vi "stage_move_absolute.vi"(7 "Stage Name":string, 8 "error in (no error)":errorcluster, 9 "wait_for_done":bool, 10 "Position":dbl, 11 "newport_xps in":refnum<class "newport_xps.lvclass">) -> (0 "error out":errorcluster, 3 "newport_xps out":refnum<class "newport_xps.lvclass">)   [LabVIEW 2015, in "newport_xps.lvclass"]
uses:
  newport_xps.lvclass
  newport_xps.lvclass/newport_xps.ctl
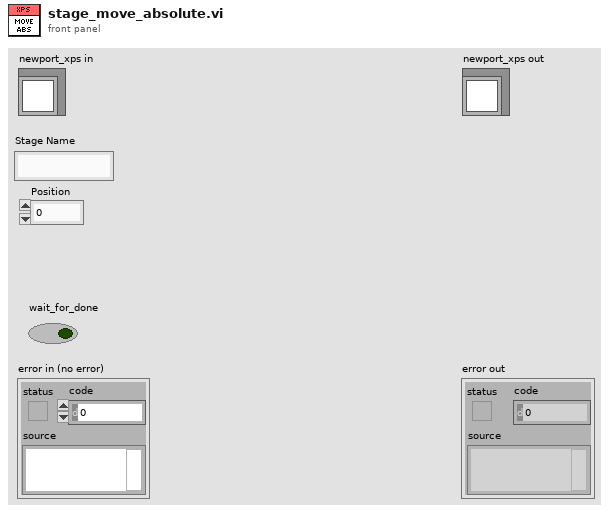
[diagram p1: front panel]
types:
  T1 = cluster{"connection TCP":refnum<k5>, "LogTo File":bool, "Log File refnum":refnum<file>, "no error if error log":bool}
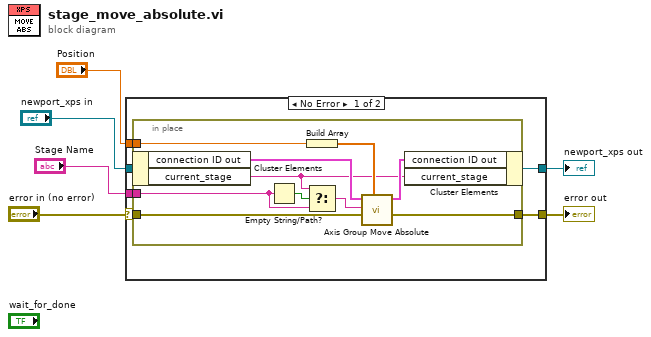
[diagram p0: block diagram]
diagram:
  n1 = case shown="No Error" "error in (no error)" {
    selector: "error in (no error)" -> [w10 w24]
    tunnel: "newport_xps in" -> [w12 w23]
    tunnel: "Stage Name" -> [w11 _]
    tunnel: "Position" -> [w9 _]
    tunnel: [w8 w24] -> w2
    tunnel: [w7 w23] -> w1
    frame No Error {
      n2 = in-place {
        in-place-border: w11 -> [w14]
        in-place-border: w10 -> [w22]
        in-place-border: w9 -> [w20]
        in-place-border: [w17] -> w8
        n3 = in-place-cluster #1(w12) -> ("connection ID out"=w21:T1, "current_stage"=w13:string)
        n4 = Empty String/Path?(string/path=w14) -> (empty?=w16:bool)
        n5 = Build Array(w20) -> (w19:dbl[])
        n6 = Select(t=w13, s=w16, f=w14) -> (s? t:f=w15:string)
        n7 = call "Axis Group Move Absolute.vi"("Target Position (units)"=w19, "XPS error in (no error)"=w22, "Group Name (250 c max)"=w15, "connection ID in"=w21) -> ("XPS error out"=w17:errorcluster, "connection ID out"=w18:T1)  [unwired: 5 in, 1 out]
        n8 = in-place-cluster #1("connection ID out"=w18, "current_stage"=w13) -> (w7:refnum<class "newport_xps.lvclass">)
      }
    }
    frame Error {
    }
  }
  "error out" <- w2
  "newport_xps out" <- w1
